vi "TEST_MCP4728.vi"() -> ()   [LabVIEW 2018]
uses:
  <vilib>/MakerHub/LINX/Private/Device/Type Defs/TCP Config.ctl
  <vilib>/MakerHub/LINX/Public/Peripherals/Digital/Digital Write 1 Chan.vi
  <vilib>/MakerHub/LINX/Public/Peripherals/Digital/Digital Write N Chans.vi
  <vilib>/MakerHub/LINX/Private/Local IO/LinxDigitalWrite.vi
  <vilib>/MakerHub/LINX/Public/Utilities/Check Channel.vi
  <vilib>/MakerHub/LINX/Public/Utilities/Open TCP.vi
  <vilib>/MakerHub/LINX/Private/Utilties/Generate Error.vi
  <vilib>/MakerHub/LINX/LMH-LINX.lvlib
  <vilib>/MakerHub/LINX/Private/Device/Device.lvlib
panel:
  in  "AUX2":enum16{"S1", "S2", "S3", "S4"}(ring)
  in  "Armed ?":bool=TRUE
  in  "Throttle (T)":u16(slide) scale=1000.0..2000.0
  in  "Yaw(R)":u16(slide) scale=1000.0..2000.0
  in  "Pitch (E)":u16(slide) scale=1000.0..2000.0
  in  "UPDATE":bool
  in  "Roll (A)":u16(slide) scale=1000.0..2000.0
  in  "UPDATE DAC":bool
  in  "INIT DAC":bool
  in  "stop":bool
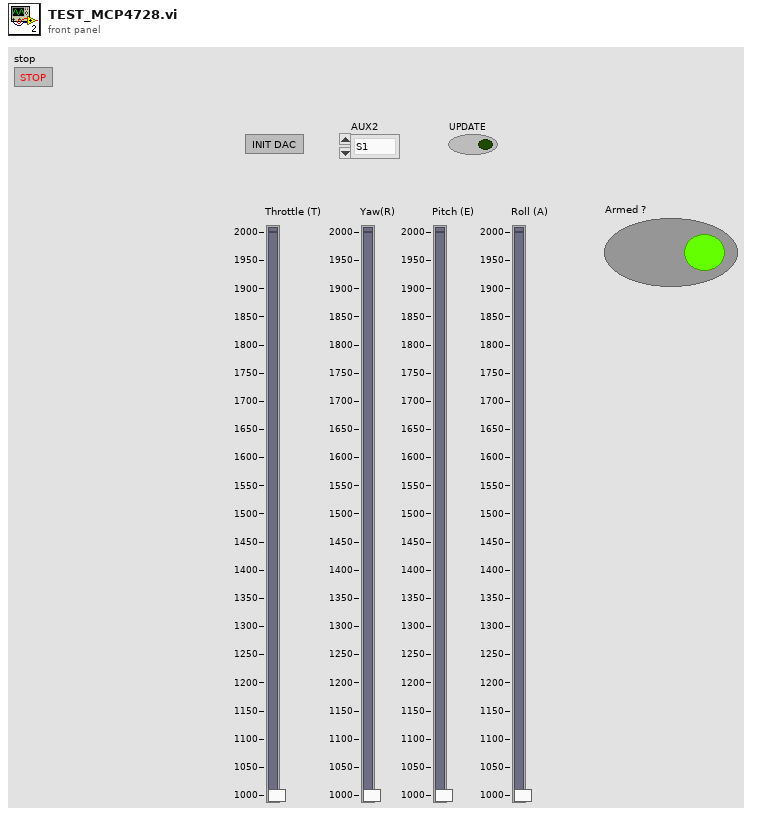
[diagram p1: front panel]
types:
  T1 = typedef "LMH-LINX.lvlib/Device.lvlib/TCP Config.ctl" = cluster{"IP Address":string, "Port":u16}
  T2 = typedef "LMH-LINX.lvlib/LINX Ref.ctl" = cluster{"IO":T3, "Interface":T4, "LINX Device Config":T5}
  T3 = typedef "LMH-LINX.lvlib/Platform.ctl" = enum16{"Remote", "Local"}
  T4 = typedef "LMH-LINX.lvlib/Interface.ctl" = enum16{"Serial", "TCP"}
  T5 = typedef "LMH-LINX.lvlib/Device.lvlib/LINX Device Config.ctl" = cluster{"Interface":T4, "COM Port":refnum<visa-resource-name>, "TCP Configuration":T1, "Device Family":u8, "Device ID":u8, "Device Name":string, "TCP Ref":refnum<k5>, "Channels":T6}
  T6 = typedef "LMH-LINX.lvlib/Channels.ctl" = cluster{"DI":u8[], "DO":u8[], "AI":u8[], "AO":u8[], "PWM":u8[], "QE":u8[], "UART":u8[], "I2C 2":u8[], "SPI":u8[], "CAN":u8[], "Servo":u8[], "AI Ref (V)":dbl, "AI Resolution (Bits)":u8, "AO Ref (V)":dbl, "AO Resolution (Bits)":u8}
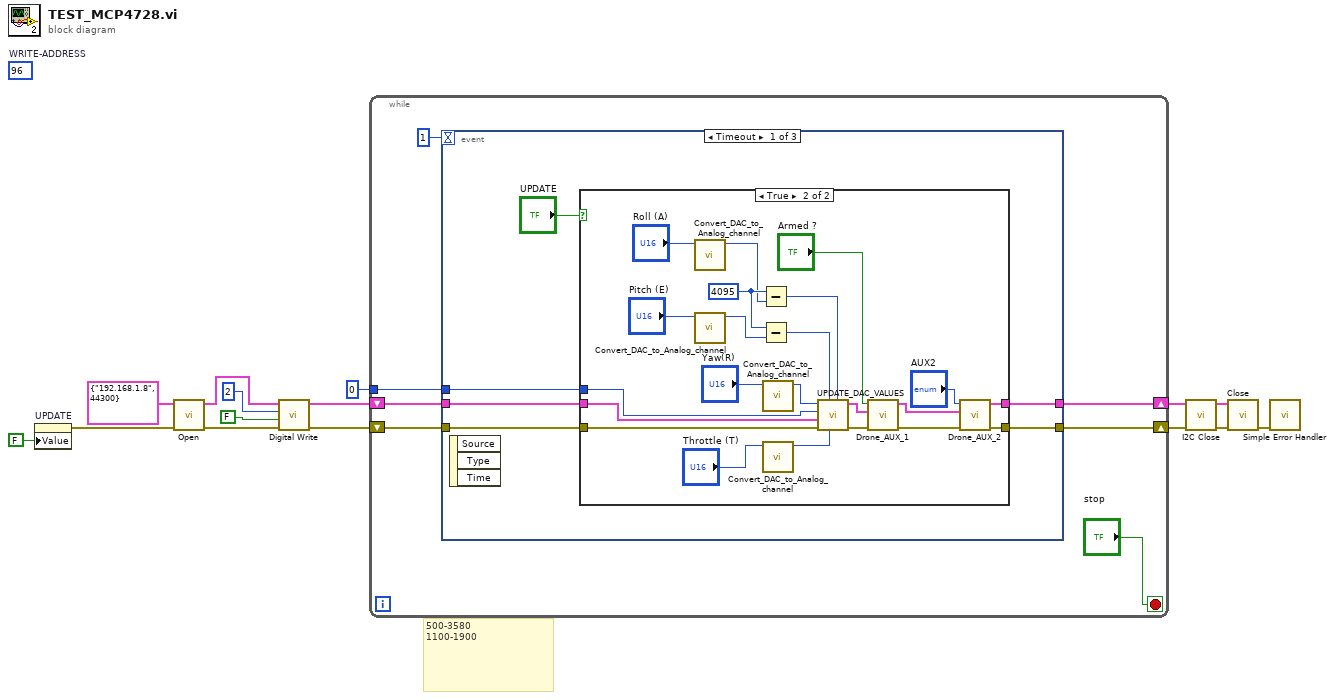
[diagram p0: block diagram]
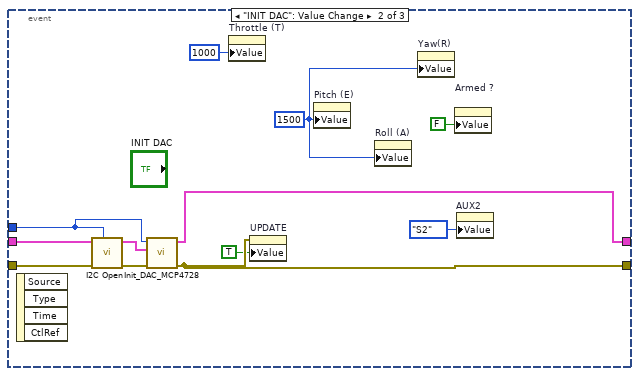
[diagram p3: hidden frame]
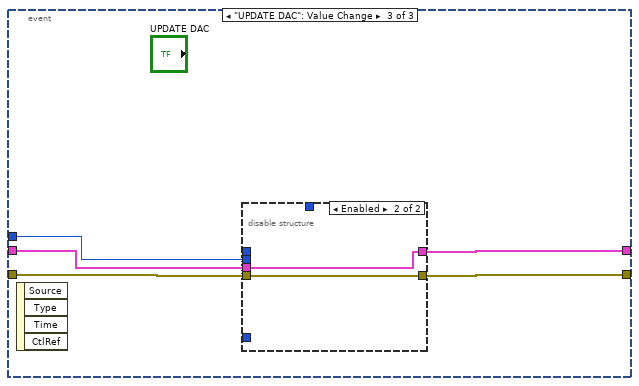
[diagram p4: hidden frame]
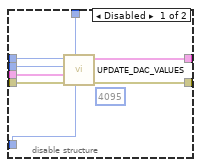
[diagram p5: hidden frame]
diagram:
  (unwired) u8 96  # WRITE-ADDRESS
  # "500-3580\n1100-1900"
  n1 = property on="UPDATE" class="Bool (strict)"("Value"=FALSE ("UPDATE")) -> (error out=w3:errorcluster)  [unwired: 2 in, 1 out]
  n2 = call-poly <vilib>:"Open.vi"("Error In"=w3, "TCP Configuration"=T1 {"IP Address"="192.168.1.8", "Port"=44300}) -> ("Error Out"=w10:errorcluster, "LINX Resource"=w12:T2)  [unwired: 7 in, 1 out]
  n3 = call-poly <vilib>:"Digital Write.vi"("Error In"=w10, "Output Value"=FALSE ("LED Value"), "DO Channel"=u8 2, "LINX Resource"=w12) -> ("Error Out"=w9:errorcluster, "LINX Resource"=w11:T2)  [unwired: 6 in]
  n4 = while {
    shift-right: [w19] -> w2
    shift-left: w11 -> [w22]
    shift-right: [w18] -> w8
    shift-left: w9 -> [w21]
    tunnel: u8 0 ("I2C Channel (0)") -> [w17]
    stop <- "stop" stop-if-true
    n5 = event shown="[0] Timeout" {
      selector: _ -> [_ _ _]
      dyn-events: _ -> [_ _ _]
      timeout: 1 -> [_ _ _]
      tunnel: w22 -> [w28 w62 w69]
      tunnel: w21 -> [w27 w61 w66]
      tunnel: [w26 w58 w65] -> w18
      tunnel: [w25 w60 w68] -> w19
      tunnel: w17 -> [w24 w59 w67]
      event Timeout {
        n6 = event-data() -> ()  [unwired: 1 in, 3 out]
        n7 = case shown="True" "UPDATE" {
          tunnel: w28 -> [w29 w52]
          tunnel: w27 -> [w30 w51]
          tunnel: [w30 w42] -> w26
          tunnel: [w29 w43] -> w25
          tunnel: w24 -> [_ w50]
          frame False {
          }
          frame True {
            w47 = u16 4095 ("x")
            n8 = call "Convert_DAC_to_Analog_channel.vi"("Analog_IN"="Roll (A)") -> ("DAC"=w38:u16)  [unwired: 10 in]
            n9 = call "Convert_DAC_to_Analog_channel.vi"("Analog_IN"="Pitch (E)") -> ("DAC"=w36:u16)  [unwired: 10 in]
            n10 = Subtract(x=w47, y=w38) -> (x-y=w46:u16)
            n11 = Subtract(x=w47, y=w36) -> (x-y=w35:u16)
            n12 = call "Convert_DAC_to_Analog_channel.vi"("Analog_IN"="Yaw(R)") -> ("DAC"=w31:u16)  [unwired: 10 in]
            n13 = call "Convert_DAC_to_Analog_channel.vi"("Analog_IN"="Throttle (T)") -> ("DAC"=w34:u16)  [unwired: 10 in]
            n14 = call "UPDATE_DAC_VALUES.vi"("A"=w46, "D"=w34, "B"=w35, "error in (no error)"=w51, "LINX Resource in"=w52, "I2C Channel (0)"=w50, "C"=w31) -> ("error out"=w45:errorcluster, "LINX Resource out"=w48:T2)  [unwired: 3 in]
            n15 = call "Drone_AUX_1.vi"("error in (no error)"=w45, "LINX Resource in"=w48, "Output Value"="Armed ?") -> ("error out"=w41:errorcluster, "LINX Resource"=w44:T2)  [unwired: 7 in]
            n16 = call "Drone_AUX_2.vi"("error in (no error)"=w41, "LINX Resource in"=w44, "AUX2"="AUX2") -> ("Error Out"=w42:errorcluster, "LINX Resource out"=w43:T2)  [unwired: 7 in]
          }
        }
      }
      event "INIT DAC": Value Change {
        w56 = u16 1500 ("Pitch (E)")
        n17 = event-data() -> ()  [unwired: 1 in, 4 out]
        n18 = call <vilib>:"I2C Open.vi"("I2C Channel (0)"=w59, "Error In"=w61, "LINX Resource"=w62) -> ("Error Out"=w63:errorcluster, "LINX Resource"=w64:T2)  [unwired: 7 in]
        n19 = call "Init_DAC_MCP4728.vi"("error in (no error)"=w63, "LINX Resource in"=w64, "I2C Channel (0)"=w59) -> ("error out"=w58:errorcluster, "LINX Resource out"=w60:T2)  [unwired: 7 in]
        n20 = property on="Throttle (T)" class="Slide (strict)"("Value"=u16 1000 ("Throttle (T)")) -> ()  [unwired: 2 in, 2 out]
        n21 = property on="UPDATE" class="Bool (strict)"(error in=w58, "Value"=TRUE ("UPDATE")) -> ()  [unwired: 1 in, 2 out]
        n22 = property on="Pitch (E)" class="Slide (strict)"("Value"=w56) -> ()  [unwired: 2 in, 2 out]
        n23 = property on="Roll (A)" class="Slide (strict)"("Value"=w56) -> ()  [unwired: 2 in, 2 out]
        n24 = property on="Yaw(R)" class="Slide (strict)"("Value"=w56) -> ()  [unwired: 2 in, 2 out]
        n25 = property on="Armed ?" class="Bool (strict)"("Value"=FALSE ("Output Value")) -> ()  [unwired: 2 in, 2 out]
        n26 = property on="AUX2" class="Enum (strict)"("Value"=enum16{"S1", "S2", "S3", "S4"}."S2" ("AUX2")) -> ()  [unwired: 2 in, 2 out]
      }
      event "UPDATE DAC": Value Change {
        n27 = event-data() -> ()  [unwired: 1 in, 4 out]
        n28 = disable-structure shown="Enabled" {
          disable-tunnel: w69 -> [w77 w79]
          disable-tunnel: [w76 w79] -> w68
          disable-tunnel: w67 -> [w75 _]
          disable-tunnel: w66 -> [w74 w78]
          disable-tunnel: [w73 w78] -> w65
          disable-tunnel: _ -> [w72 _]
          disable-tunnel: _ -> [w71 _]
          disable-tunnel: _ -> [w70 _]
          frame Disabled {
            (unwired) 4095
            n29 = call "UPDATE_DAC_VALUES.vi"("D"=w70, "B"=w72, "error in (no error)"=w74, "LINX Resource in"=w77, "I2C Channel (0)"=w75, "C"=w71) -> ("error out"=w73:errorcluster, "LINX Resource out"=w76:T2)  [unwired: 4 in]
          }
          frame Enabled {
          }
        }
      }
    }
  }
  n30 = call <vilib>:"I2C Close.vi"("Error In"=w8, "LINX Resource"=w2) -> ("Error Out"=w7:errorcluster, "LINX Resource"=w6:T2)  [unwired: 8 in]
  n31 = call <vilib>:"Close.vi"("Error In"=w7, "LINX Resource"=w6) -> ("Error Out"=w1:errorcluster)  [unwired: 9 in]
  n32 = call <vilib>:"Simple Error Handler.vi"("error in (no error)"=w1) -> ()  [unwired: 4 in, 5 out]
